vi "Common Configuration.vi"(0 "Instrument Handle In":refnum<k21>, 1 "Selector String":string, 5 "Common Configuration":T5={"Measurement Interval (s)"=0.0001, "Signal Type"=0, "DUT Average Input Power (dBm)"=-15.0, "Synchronization Method"=1} {"Synchronization Method" items=["False", "True"]; "DUT Average Input Power (dBm)" format="%.2f"; "Signal Type" items=["Modulated", "Tones"]; "Measurement Interval (s)" format="%#.2p"}, 7 "Pre-DPD CFR":T4={"CFR Enabled"=0, "CFR Method"=0, "Max Iterations"=10, "Target PAPR (dB)"=8.0, "Peak Windowing"={"Window Type"=7, "Window Length"=10}, "Sigmoid"={"Shaping Factor"=5.0, "Shaping Threshold (dB)"=-5.0}, "Filter Enabled"=0, "Signal Settings"={"Carrier Offsets (Hz)"=[0.0], "Carrier Bandwidths (Hz)"=[20000000.0]}} {"Signal Settings"."Carrier Bandwidths (Hz)" format="%.2p"; "Signal Settings"."Carrier Offsets (Hz)" format="%.2p"; "Filter Enabled" items=["False", "True"]; "Peak Windowing"."Window Type" items=["Flat Top"=1, "Hanning"=2, "Hamming"=3, "Gaussian"=4, "Blackman"=5, "Blackman-Harris"=6, "Kaiser-Bessel"=7]; "CFR Method" items=["Clipping", "Peak Windowing", "Sigmoid"]; "CFR Enabled" items=["False", "True"]}, 9 "Waveform":T1={"Waveform Name"="Wfm", "Waveform"={"x0"=0.0, "dx"=0.0, "y"=[]}, "Signal Bandwidth (Hz)"=0.0, "PAPR (dB)"=0.0, "Burst Length (s)"=0.0, "Sample Rate"=0.0, "Burst Start Locations"=[], "Burst Stop Locations"=[], "Idle Duration Present?"=FALSE, "Runtime Scaling"=0.0} {"Runtime Scaling" format="%#_6p"; "Sample Rate" format="%#_6p"; "Burst Length (s)" format="%#_6p"; "PAPR (dB)" format="%.2f"; "Signal Bandwidth (Hz)" format="%#_6p"; "Waveform"."y" format="%.2f"; "Waveform"."dx" format="%^.2e"; "Waveform"."x0" format="%^.2e"}, 11 "error in (no error)":errorcluster, 12 "Apply DPD CFR":T3={"CFR Enabled"=0, "CFR Method"=0, "Max Iterations"=10, "Target PAPR Type"=0, "Target PAPR (dB)"=8.0, "Peak Windowing"={"Window Type"=7, "Window Length"=10}, "Sigmoid"={"Shaping Factor"=5.0, "Shaping Threshold (dB)"=-5.0}} {"Target PAPR Type" items=["Input PAPR", "Custom"]; "Peak Windowing"."Window Type" items=["Flat Top"=1, "Hanning"=2, "Hamming"=3, "Gaussian"=4, "Blackman"=5, "Blackman-Harris"=6, "Kaiser-Bessel"=7]; "CFR Method" items=["Clipping", "Peak Windowing", "Sigmoid"]; "CFR Enabled" items=["False", "True"]}) -> (4 "Instrument Handle Out":refnum<k21>, 6 "Pre DPD CFR Waveform Out":T2={"Waveform Name"="Wfm", "Waveform"={"x0"=0.0, "dx"=0.0, "y"=[]}, "Signal Bandwidth (Hz)"=0.0, "PAPR (dB)"=0.0, "Burst Length (s)"=0.0, "Sample Rate"=0.0, "Burst Start Locations"=[], "Burst Stop Locations"=[], "Idle Duration Present?"=FALSE, "Runtime Scaling"=0.0} {"Runtime Scaling" format="%#_6p"; "Sample Rate" format="%#_6p"; "Burst Length (s)" format="%#_6p"; "PAPR (dB)" format="%.2f"; "Signal Bandwidth (Hz)" format="%#_6p"; "Waveform"."y" format="%.2f"; "Waveform"."dx" format="%^.2e"; "Waveform"."x0" format="%^.2e"}, 15 "error out":errorcluster)   [LabVIEW 2016, in "RFmxDPD.lvlib"]
uses:
  RFmxDPD.lvlib
  Typedefs/Common Configuration.ctl
  Typedefs/Pre DPD CFR.ctl
  Typedefs/Apply DPD CFR.ctl
  SG/Typedefs/Waveform.ctl
  <vilib>/RFmx/SpecAn/mx/RFmxSpecAn.llb/RFmxSpecAn Select Measurement (Single).vi
  <resource>/objmgr/RFmxSpecAn.rc
  SG/SG.lvlib
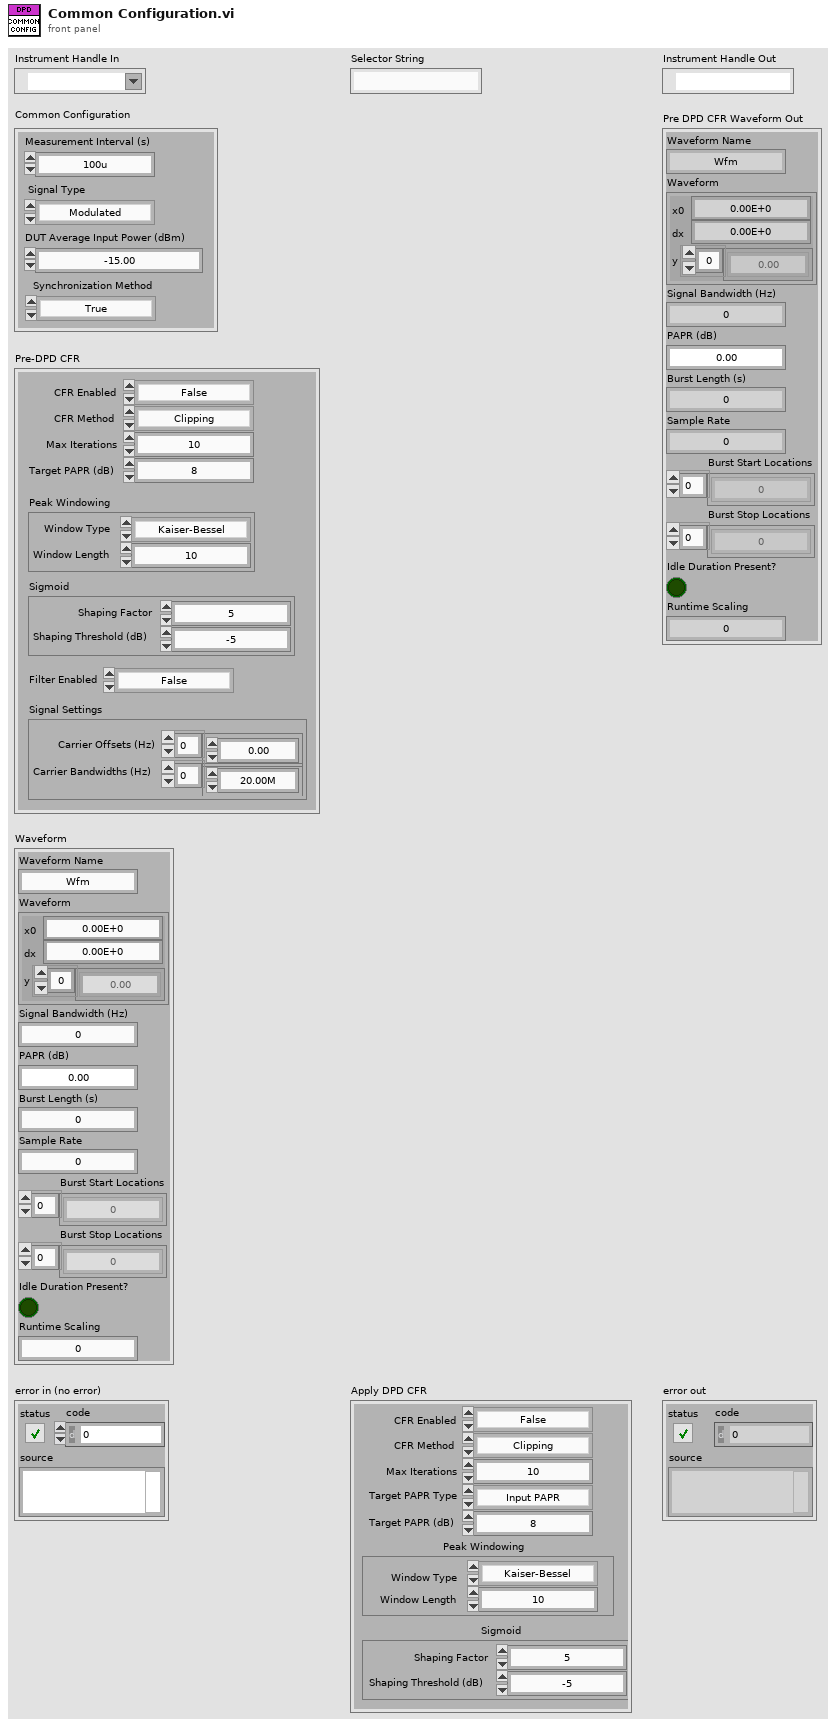
[diagram p1: front panel]
types:
  T1 = typedef "SG.lvlib/Waveform.ctl" = cluster{"Waveform Name":string, "Waveform":cluster{"x0":dbl, "dx":dbl, "y":csg[]}, "Signal Bandwidth (Hz)":dbl, "PAPR (dB)":dbl, "Burst Length (s)":dbl, "Sample Rate":dbl, "Burst Start Locations":i32[], "Burst Stop Locations":i32[], "Idle Duration Present?":bool, "Runtime Scaling":dbl}
  T2 = cluster{"Waveform Name":string, "Waveform":cluster{"x0":dbl, "dx":dbl, "y":csg[]}, "Signal Bandwidth (Hz)":dbl, "PAPR (dB)":dbl, "Burst Length (s)":dbl, "Sample Rate":dbl, "Burst Start Locations":i32[], "Burst Stop Locations":i32[], "Idle Duration Present?":bool, "Runtime Scaling":dbl}
  T3 = typedef "RFmxDPD.lvlib/Apply DPD CFR.ctl" = cluster{"CFR Enabled":i32, "CFR Method":i32, "Max Iterations":i32, "Target PAPR Type":i32, "Target PAPR (dB)":dbl, "Peak Windowing":cluster{"Window Type":i32, "Window Length":i32}, "Sigmoid":cluster{"Shaping Factor":dbl, "Shaping Threshold (dB)":dbl}}
  T4 = typedef "RFmxDPD.lvlib/Pre DPD CFR.ctl" = cluster{"CFR Enabled":i32, "CFR Method":i32, "Max Iterations":i32, "Target PAPR (dB)":dbl, "Peak Windowing":cluster{"Window Type":i32, "Window Length":i32}, "Sigmoid":cluster{"Shaping Factor":dbl, "Shaping Threshold (dB)":dbl}, "Filter Enabled":i32, "Signal Settings":cluster{"Carrier Offsets (Hz)":dbl[], "Carrier Bandwidths (Hz)":dbl[]}}
  T5 = typedef "RFmxDPD.lvlib/Common Configuration.ctl" = cluster{"Measurement Interval (s)":dbl, "Signal Type":i32, "DUT Average Input Power (dBm)":dbl, "Synchronization Method":i32}
  T6 = enum16{"ACP", "CCDF", "CHP", "FCnt", "Harmonics", "OBW", "SEM", "Spectrum", "Spur", "TXP", "AMPM", "DPD", "IQ", "IM", "NF", "PhaseNoise"}
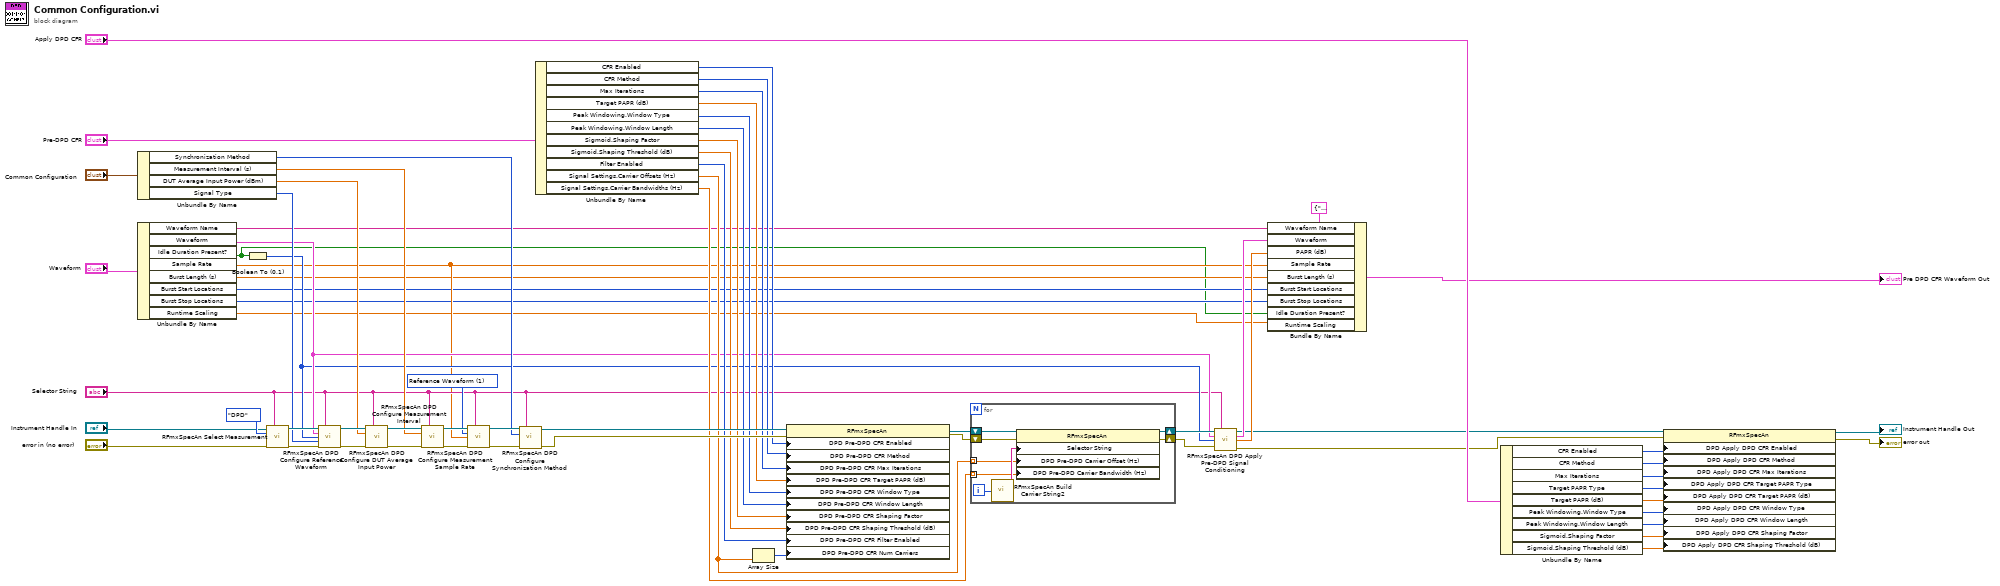
[diagram p0: block diagram]
diagram:
  w53 = 1 items=["User", "Reference Waveform"] ("Sample Rate Mode")
  n1 = Unbundle By Name("Common Configuration") -> ("Synchronization Method"=w50:i32, "Measurement Interval (s)"=w54:dbl, "DUT Average Input Power (dBm)"=w55:dbl, "Signal Type"=w56:i32)
  n2 = Unbundle By Name("Waveform") -> ("Waveform Name"=w12:string, "Waveform"=w17:cluster{"x0":dbl, "dx":dbl, "y":csg[]}, "Idle Duration Present?"=w5:bool, "Sample Rate"=w9:dbl, "Burst Length (s)"=w8:dbl, "Burst Start Locations"=w7:i32[], "Burst Stop Locations"=w6:i32[], "Runtime Scaling"=w4:dbl)
  n3 = Boolean To (0,1)(Boolean=w5) -> (0, 1=w16:i16)
  n4 = call-poly <vilib>:"RFmxSpecAn Select Measurement.vi"("Instrument Handle In"="Instrument Handle In", "Selector String"="Selector String", "Measurement"=T6."DPD", "error in (no error)"="error in (no error)") -> ("Instrument Handle Out"=w64:refnum<k21>, "error out"=w63:errorcluster)  [unwired: 10 in]
  n5 = call <vilib>:"RFmxSpecAn DPD Configure Reference Waveform.vi"("Instrument Handle In"=w64, "Selector String"="Selector String", "Reference Waveform"=w17, "Idle Duration Present"=w16, "Signal Type"=w56, "error in (no error)"=w63) -> ("Instrument Handle Out"=w62:refnum<k21>, "error out"=w61:errorcluster)  [unwired: 8 in]
  n6 = call <vilib>:"RFmxSpecAn DPD Configure DUT Average Input Power.vi"("Instrument Handle In"=w62, "Selector String"="Selector String", "DUT Average Input Power (dBm)"=w55, "error in (no error)"=w61) -> ("Instrument Handle Out"=w60:refnum<k21>, "error out"=w59:errorcluster)  [unwired: 10 in]
  n7 = call <vilib>:"RFmxSpecAn DPD Configure Measurement Interval.vi"("Instrument Handle In"=w60, "Selector String"="Selector String", "Measurement Interval (s)"=w54, "error in (no error)"=w59) -> ("Instrument Handle Out"=w58:refnum<k21>, "error out"=w57:errorcluster)  [unwired: 10 in]
  n8 = call <vilib>:"RFmxSpecAn DPD Configure Measurement Sample Rate.vi"("Instrument Handle In"=w58, "Selector String"="Selector String", "Sample Rate Mode"=w53, "Sample Rate (S/s)"=w9, "error in (no error)"=w57) -> ("Instrument Handle Out"=w52:refnum<k21>, "error out"=w51:errorcluster)  [unwired: 9 in]
  n9 = call <vilib>:"RFmxSpecAn DPD Configure Synchronization Method.vi"("Instrument Handle In"=w52, "Selector String"="Selector String", "Synchronization Method"=w50, "error in (no error)"=w51) -> ("Instrument Handle Out"=w45:refnum<k21>, "error out"=w44:errorcluster)  [unwired: 10 in]
  n10 = Unbundle By Name("Pre-DPD CFR") -> ("CFR Enabled"=w33:i32, "CFR Method"=w32:i32, "Max Iterations"=w31:i32, "Target PAPR (dB)"=w30:dbl, "Peak Windowing.Window Type"=w29:i32, "Peak Windowing.Window Length"=w28:i32, "Sigmoid.Shaping Factor"=w27:dbl, "Sigmoid.Shaping Threshold (dB)"=w26:dbl, "Filter Enabled"=w25:i32, "Signal Settings.Carrier Offsets (Hz)"=w24:dbl[], "Signal Settings.Carrier Bandwidths (Hz)"=w23:dbl[])
  n11 = Array Size(array=w24) -> (size(s)=w46:i32)
  n12 = property class="RFmxSpecAn"(reference=w45, error in=w44, "DPD Pre-DPD CFR Enabled"=w33, "DPD Pre-DPD CFR Method"=w32, "DPD Pre-DPD CFR Max Iterations"=w31, "DPD Pre-DPD CFR Target PAPR (dB)"=w30, "DPD Pre-DPD CFR Window Type"=w29, "DPD Pre-DPD CFR Window Length"=w28, "DPD Pre-DPD CFR Shaping Factor"=w27, "DPD Pre-DPD CFR Shaping Threshold (dB)"=w26, "DPD Pre-DPD CFR Filter Enabled"=w25, "DPD Pre-DPD CFR Num Carriers"=w46) -> (reference out=w47:refnum<k21>, error out=w48:errorcluster)
  n13 = for {
    shift-right: [w74] -> w18
    shift-left: w48 -> [w75]
    shift-right: [w72] -> w19
    shift-left: w47 -> [w73]
    tunnel: w24 -> [w69] mode=indexing
    tunnel: w23 -> [w68] mode=indexing
    i -> [w71]
    n14 = call <vilib>:"RFmxSpecAn Build Carrier String2.vi"("Carrier Number"=w71) -> ("Selector String Out"=w70:string)  [unwired: 14 in]
    n15 = property class="RFmxSpecAn"(reference=w73, error in=w75, "Selector String"=w70, "DPD Pre-DPD Carrier Offset (Hz)"=w69, "DPD Pre-DPD Carrier Bandwidth (Hz)"=w68) -> (reference out=w72:refnum<k21>, error out=w74:errorcluster)
  }
  n16 = call <vilib>:"RFmxSpecAn DPD Apply Pre-DPD Signal Conditioning.vi"("Instrument Handle In"=w19, "Selector String"="Selector String", "Waveform In"=w17, "Idle Duration Present"=w16, "error in (no error)"=w18) -> ("Instrument Handle Out"=w3:refnum<k21>, "Waveform Out"=w11:cluster{"x0":dbl, "dx":dbl, "y":csg[]}, "PAPR (dB)"=w10:dbl, "error out"=w2:errorcluster)  [unwired: 7 in]
  n17 = Bundle By Name(cluster=T2 {"Waveform Name"="Wfm", "Waveform"={"x0"=0.0, "dx"=0.0, "y"=[]}, "Signal Bandwidth (Hz)"=0.0, "PAPR (dB)"=0.0, "Burst Length (s)"=0.0, "Sample Rate"=0.0, "Burst Start Locations"=[], "Burst Stop Locations"=[], "Idle Duration Present?"=FALSE, "Runtime Scaling"=0.0} ("Waveform Out"), "Waveform Name"=w12, "Waveform"=w11, "PAPR (dB)"=w10, "Sample Rate"=w9, "Burst Length (s)"=w8, "Burst Start Locations"=w7, "Burst Stop Locations"=w6, "Idle Duration Present?"=w5, "Runtime Scaling"=w4) -> (→"Pre DPD CFR Waveform Out":T2)
  n18 = Unbundle By Name("Apply DPD CFR") -> ("CFR Enabled"=w36:i32, "CFR Method"=w37:i32, "Max Iterations"=w38:i32, "Target PAPR Type"=w35:i32, "Target PAPR (dB)"=w39:dbl, "Peak Windowing.Window Type"=w40:i32, "Peak Windowing.Window Length"=w41:i32, "Sigmoid.Shaping Factor"=w42:dbl, "Sigmoid.Shaping Threshold (dB)"=w43:dbl)
  n19 = property class="RFmxSpecAn"(reference=w3, error in=w2, "DPD Apply DPD CFR Enabled"=w36, "DPD Apply DPD CFR Method"=w37, "DPD Apply DPD CFR Max Iterations"=w38, "DPD Apply DPD CFR Target PAPR Type"=w35, "DPD Apply DPD CFR Target PAPR (dB)"=w39, "DPD Apply DPD CFR Window Type"=w40, "DPD Apply DPD CFR Window Length"=w41, "DPD Apply DPD CFR Shaping Factor"=w42, "DPD Apply DPD CFR Shaping Threshold (dB)"=w43) -> (reference out=→"Instrument Handle Out":refnum<k21>, error out=→"error out":errorcluster)
